vi "JSONFlatternAndUnflatten.vi"() -> ()   [LabVIEW 2020]
panel:
  out "Employee 2":cluster{"Name":string, "Age":u8, "Salary":u32}
  in  "JSON string 2":string
  out "JSON string":string
  in  "Employee":cluster{"Name":string, "Age":u8, "Salary":u32}
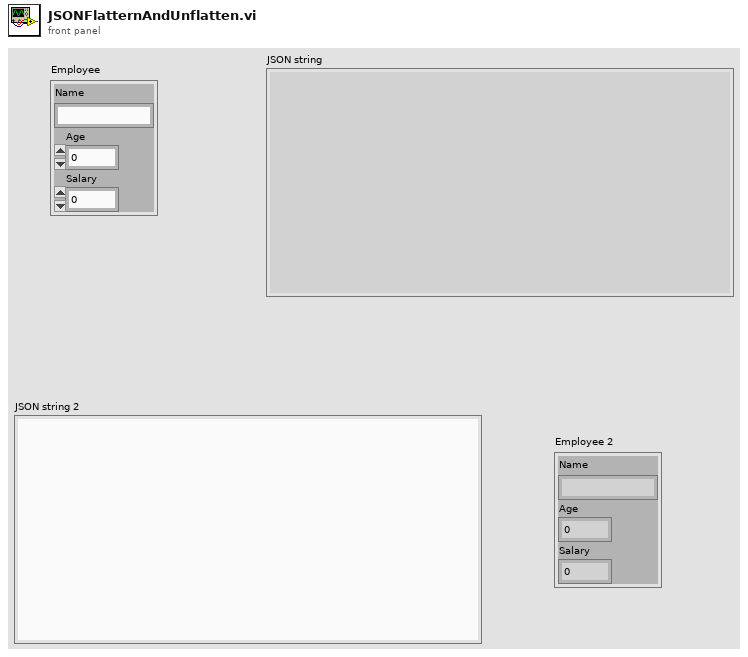
[diagram p1: front panel]
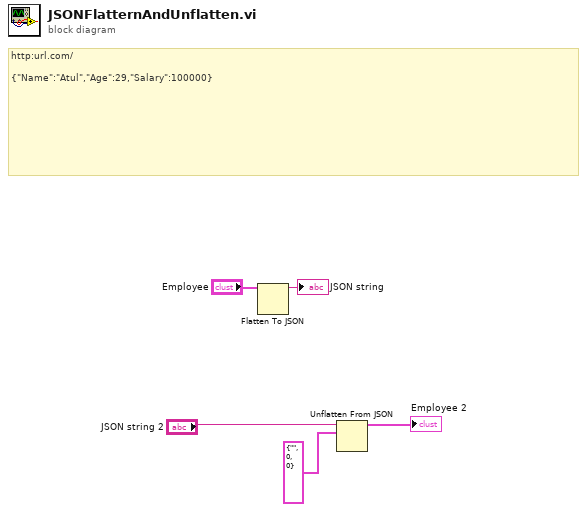
[diagram p0: block diagram]
diagram:
  # "http:url.com/\n\n{\"Name\":\"Atul\",\"Age\":29,\"Salary\":100000}"
  n1 = Flatten To JSON(anything="Employee") -> (JSON string=→"JSON string":string)  [unwired: 2 in, 1 out]
  n2 = Unflatten From JSON(JSON string="JSON string 2", type and defaults=cluster{"Name":string, "Age":u8, "Salary":u32} {"Name"="", "Age"=0, "Salary"=0} ("Employee 2")) -> (value=→"Employee 2":cluster{"Name":string, "Age":u8, "Salary":u32})  [unwired: 5 in, 1 out]
